vi "write_attributes.vi"(8 "error in (no error)":errorcluster, 10 "attributes":T1, 11 "IncrementalPCA in":refnum<class "IncrementalPCA.lvclass">) -> (0 "error out":errorcluster, 3 "IncrementalPCA out":refnum<class "IncrementalPCA.lvclass">)   [LabVIEW 2020, in "IncrementalPCA.lvclass"]
uses:
  IncrementalPCA.lvclass
  Controls/incremental_pca_attributes.ctl
  IncrementalPCA.lvclass/IncrementalPCA.ctl
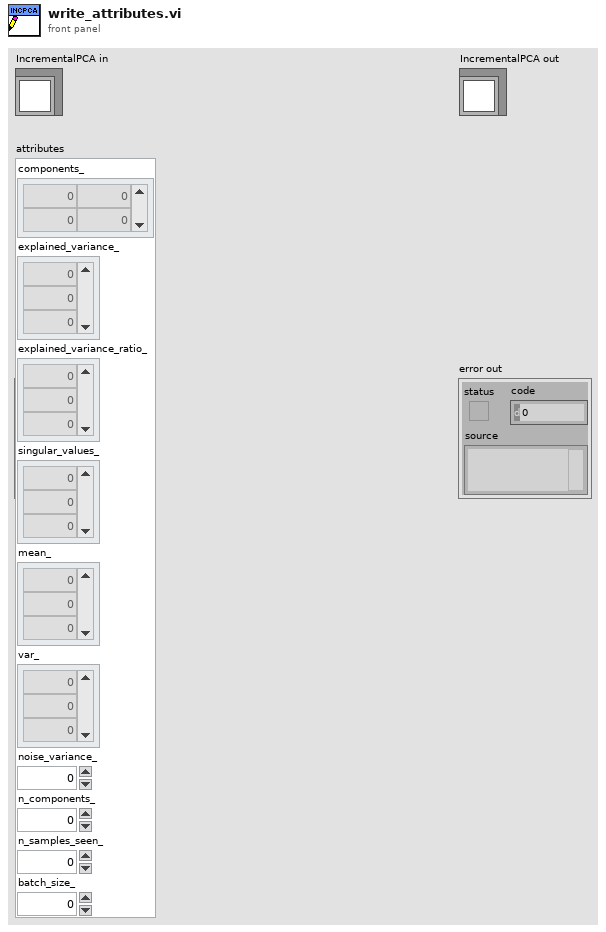
[diagram p1: front panel]
types:
  T1 = typedef "incremental_pca_attributes.ctl" = cluster{"components_":dbl[][], "explained_variance_":dbl[], "explained_variance_ratio_":dbl[], "singular_values_":dbl[], "mean_":dbl[], "var_":dbl[], "noise_variance_":dbl, "n_components_":dbl, "n_samples_seen_":dbl, "batch_size_":dbl}
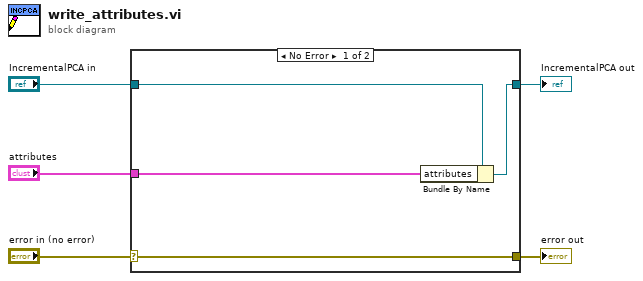
[diagram p0: block diagram]
diagram:
  n1 = case shown="No Error" "error in (no error)" {
    selector: "error in (no error)" -> [w9 w10]
    tunnel: [w9 w10] -> w4
    tunnel: [w7 w11] -> w2
    tunnel: "IncrementalPCA in" -> [w8 w11]
    tunnel: "attributes" -> [w6 _]
    frame No Error {
      n2 = Bundle By Name(cluster=w8, "attributes"=w6) -> (w7:refnum<class "IncrementalPCA.lvclass">)
    }
    frame Error {
    }
  }
  "error out" <- w4
  "IncrementalPCA out" <- w2
